vi "20150818 Combined test.vi"() -> ()   [LabVIEW 2013]
panel:
  out "Error Out":errorcluster
  in  "stop":bool
  in  "Pulse Widths (uS)":u16[](array[numeric])=[1500, 1500, 1500, 1500, 1500, 1500, 1500, 1500, 1500, 1500, 1500, 1500] min=600 max=2400 step=100
  out "Distance(cm)":dbl
  out "Servo initialize OK?":bool
  out "UL sensor initialize OK?":bool
  in  "Serial Port":refnum<visa-resource-name>="COM10"
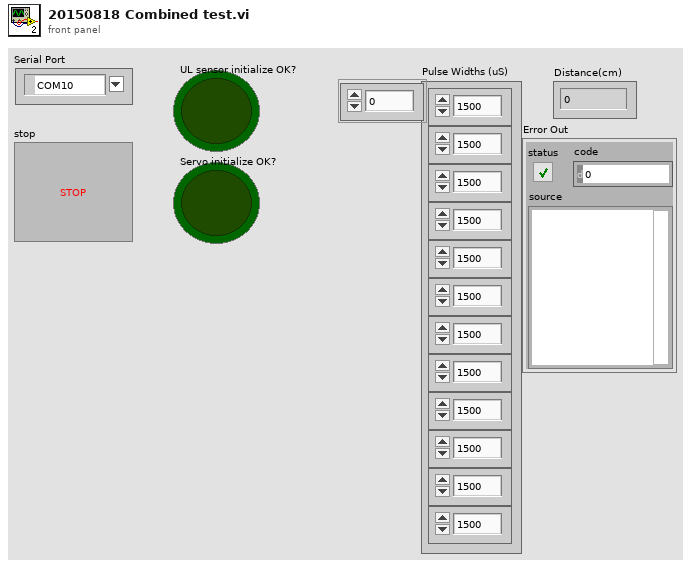
[diagram p1: front panel]
types:
  T1 = enum16{"Initialize", "Close", "Set Pulse widths"}
  T2 = typedef "LMH-LINX.lvlib/LINX Ref.ctl" = cluster{"Platform":T3, "Interface":T4, "LINX Device Config":T5}
  T3 = typedef "LMH-LINX.lvlib/Platform.ctl" = enum16{"LINX", "myRIO"}
  T4 = typedef "LMH-LINX.lvlib/Interface.ctl" = enum16{"Serial", "TCP"}
  T5 = typedef "LMH-LINX.lvlib/Device.lvlib/LINX Device Config.ctl" = cluster{"Interface":T4, "COM Port":refnum<visa-resource-name>, "TCP Configuration":T6, "Device Family":u8, "Device ID":u8, "Device Name":string, "TCP Ref":refnum<k5>, "Channels":T7}
  T6 = typedef "LMH-LINX.lvlib/Device.lvlib/TCP Config.ctl" = cluster{"IP Address":string, "Port":u16}
  T7 = typedef "LMH-LINX.lvlib/Channels.ctl" = cluster{"DI":u8[], "DO":u8[], "AI":u8[], "AO":u8[], "PWM":u8[], "QE":u8[], "UART":u8[], "I2C 2":u8[], "SPI":u8[], "CAN":u8[], "Servo":u8[], "AI Ref (V)":dbl, "AO Ref (V)":dbl, "AO Resolution (Bits)":u8}
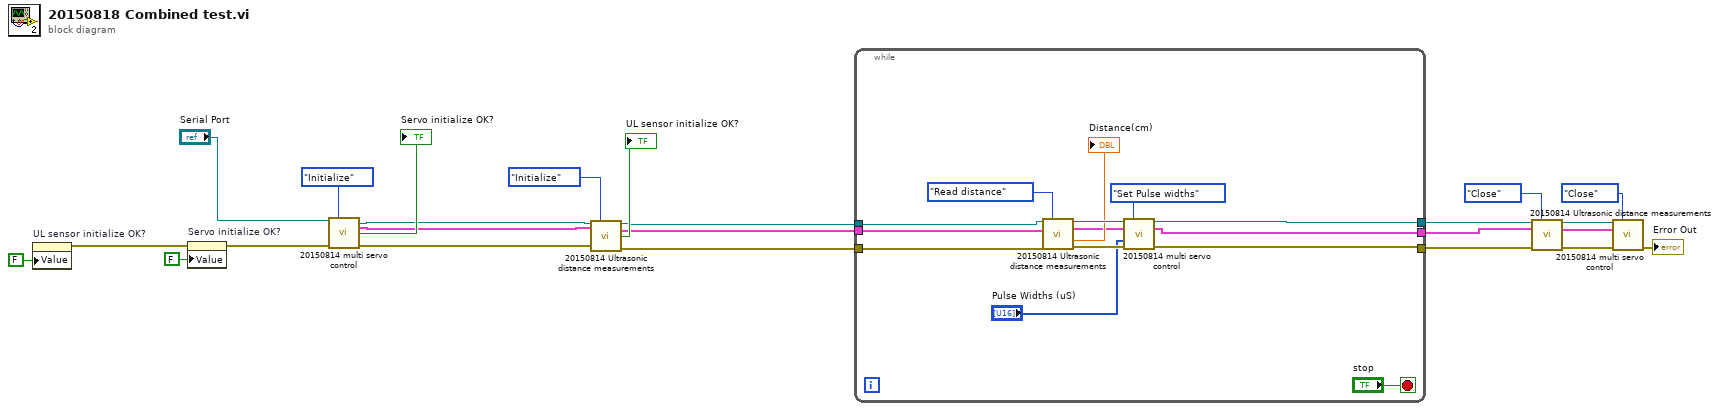
[diagram p0: block diagram]
diagram:
  n1 = property on="UL sensor initialize OK?" class="Bool (strict)"("Value"=FALSE ("UL sensor initialize OK?")) -> (error out=w17:errorcluster)  [unwired: 2 in, 1 out]
  n2 = property on="Servo initialize OK?" class="Bool (strict)"(error in=w17, "Value"=FALSE ("Servo initialize OK?")) -> (error out=w8:errorcluster)  [unwired: 1 in, 1 out]
  n3 = call "20150814 multi servo control.vi"("Serial Port"="Serial Port", "Action"=T1."Initialize", "error in (no error)"=w8) -> ("Serial Port out"=w2:refnum<visa-resource-name>, "LINX Resource out"=w3:T2, "Servo initialize OK?"=→"Servo initialize OK?":bool, "Error Out"=w7:errorcluster)  [unwired: 9 in]
  n4 = call "20150814 Ultrasonic distance measurements.vi"("Serial Port"=w2, "Action"=enum16{"Initialize", "Close", "Read distance"}."Initialize", "LINX Resource in"=w3, "error in (no error)"=w7) -> ("Serial Port out"=w5:refnum<visa-resource-name>, "LINX Resource out"=w4:T2, "UL sensor initialize OK?"=→"UL sensor initialize OK?":bool, "Error Out"=w6:errorcluster)  [unwired: 7 in, 1 out]
  n5 = while {
    tunnel: w6 -> [w37]
    tunnel: [w36] -> w21
    tunnel: w5 -> [w35]
    tunnel: [w33] -> w20
    tunnel: w4 -> [w27]
    tunnel: [w25] -> w14
    stop <- "stop" stop-if-true
    n6 = call "20150814 Ultrasonic distance measurements.vi"("Serial Port"=w35, "Action"=enum16{"Initialize", "Close", "Read distance"}."Read distance", "LINX Resource in"=w27, "error in (no error)"=w37) -> ("Serial Port out"=w34:refnum<visa-resource-name>, "LINX Resource out"=w26:T2, "Distance(cm)"=→"Distance(cm)":dbl, "Error Out"=w38:errorcluster)  [unwired: 7 in, 1 out]
    n7 = call "20150814 multi servo control.vi"("Serial Port"=w34, "Action"=T1."Set Pulse widths", "LINX Resource in"=w26, "Pulse Widths (uS)"="Pulse Widths (uS)", "error in (no error)"=w38) -> ("Serial Port out"=w33:refnum<visa-resource-name>, "LINX Resource out"=w25:T2, "Error Out"=w36:errorcluster)  [unwired: 7 in, 1 out]
  }
  n8 = call "20150814 Ultrasonic distance measurements.vi"("Serial Port"=w20, "Action"=enum16{"Initialize", "Close", "Read distance"}."Close", "LINX Resource in"=w14, "error in (no error)"=w21) -> ("Serial Port out"=w19:refnum<visa-resource-name>, "LINX Resource out"=w13:T2, "Error Out"=w22:errorcluster)  [unwired: 7 in, 2 out]
  n9 = call "20150814 multi servo control.vi"("Serial Port"=w19, "Action"=T1."Close", "LINX Resource in"=w13, "error in (no error)"=w22) -> ("Error Out"=→"Error Out":errorcluster)  [unwired: 8 in, 3 out]
